vi "dcimgToTif.vi"(1 "flattenedFilenamesArray":path[](array[path])) -> (0 "conversionComplete?":bool)   [LabVIEW 2015]
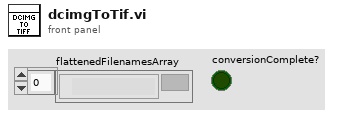
[diagram p1: front panel]
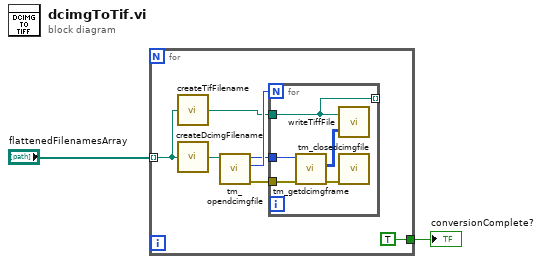
[diagram p0: block diagram]
diagram:
  n1 = for {
    tunnel: "flattenedFilenamesArray" -> [w4] mode=indexing
    tunnel: [TRUE ("conversionComplete?")] -> w1
    n2 = call "createTifFilename.vi"("inputPath"=w4) -> ("tifPath"=w5:path)
    n3 = call "createDcimgFilename.vi"("origPath"=w4) -> ("dcimgPath"=w3:path)
    n4 = call <userlib>:"tm_opendcimgfile.vi"("Path"=w3) -> ("error out"=w7:errorcluster, "Total Frames"=w9:i32, "File Handle"=w8:u32)  [unwired: 8 in]
    n5 = for {
      N: w9 -> [_]
      tunnel: w5 -> [w10]
      tunnel: w8 -> [w13]
      tunnel: w7 -> [w12]
      tunnel: [w10] -> _ mode=indexing
      n6 = call <userlib>:"tm_getdcimgframe.vi"("error in (no error)"=w12, "File Handle in"=w13) -> ("error out"=w11:errorcluster, "Data"=w14:u16[][])  [unwired: 6 in, 2 out]
      n7 = call "writeTiffFile.vi"("Image Pixels (U16)"=w14, "File Path"=w10) -> ()
      n8 = call <userlib>:"tm_closedcimgfile.vi"("error in (no error)"=w11) -> ()  [unwired: 10 in, 1 out]
    }
  }
  "conversionComplete?" <- w1
